vi "Get Session Cookie.vi"() -> (3 "Session":string)   [LabVIEW 2021]
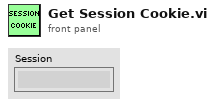
[diagram p1: front panel]
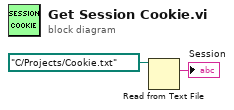
[diagram p0: block diagram]
diagram:
  n1 = Read from Text File(file (use dialog)=path "C:/Projects/Cookie.txt") -> (text=→"Session":string)  [unwired: 3 in, 3 out]
